vi "GEM_BANK_ARRAY_Flatten.vi"(8 "error in (no error)":errorcluster, 11 "LVBANKARRAY in":refnum<class "GEM_BANK_ARRAY.lvclass">) -> (0 "error out":errorcluster, 2 "Array":u8[](array[numeric]), 3 "LVBANKARRAY out":refnum<class "GEM_BANK_ARRAY.lvclass">)   [LabVIEW 2018, in "feGEM DataPacker.lvlib" / "GEM_BANK_ARRAY.lvclass"]
uses:
  GEM_BANK_ARRAY.lvclass
  GEM_BANK_ARRAY.lvclass/GEM_BANK_ARRAY.ctl
  GEM_BANK.lvclass
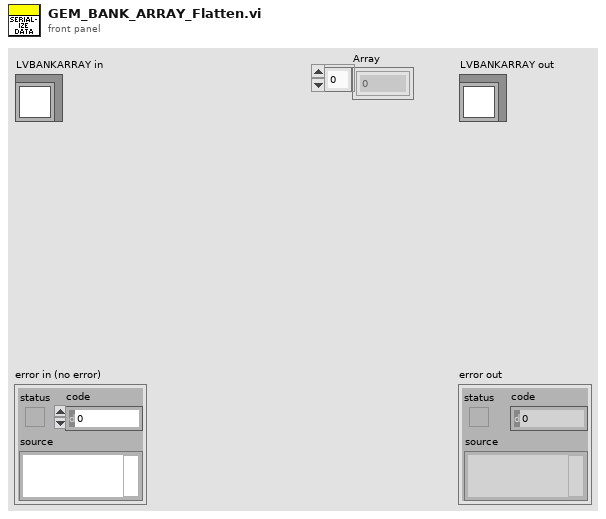
[diagram p1: front panel]
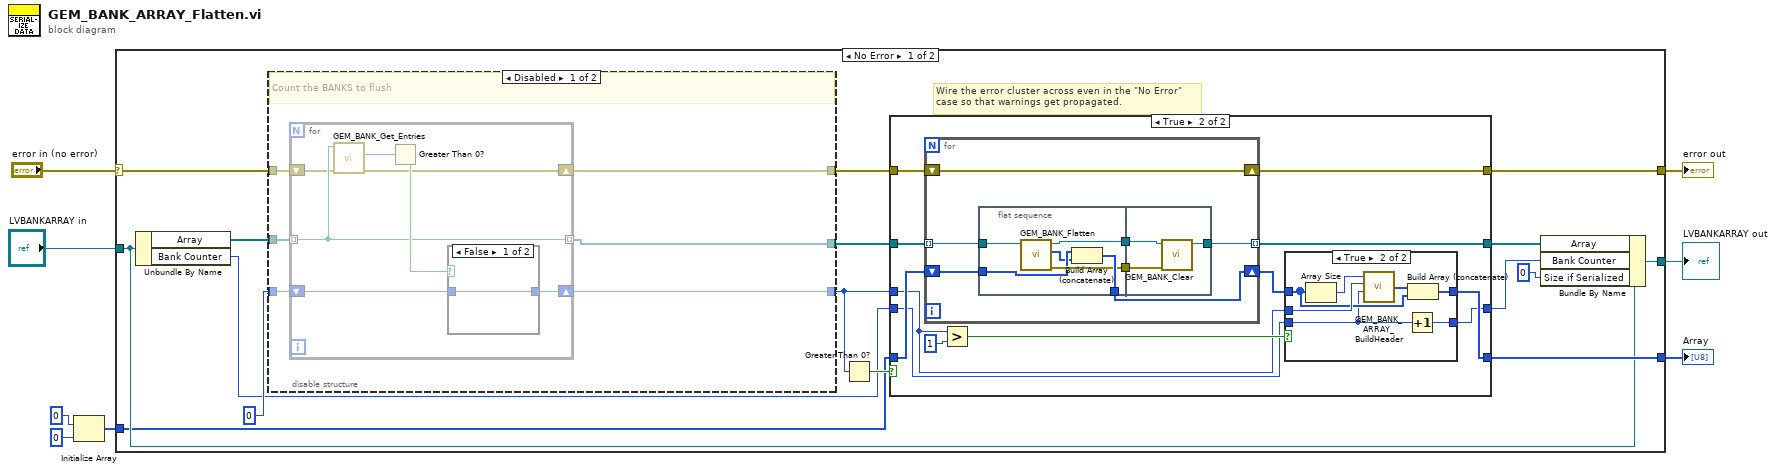
[diagram p0: block diagram]
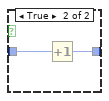
[diagram p2: hidden frame]
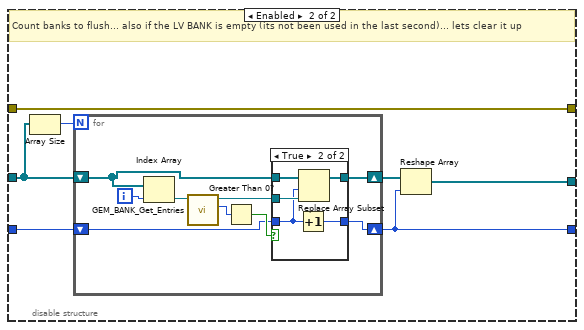
[diagram p3: hidden frame]
diagram:
  n1 = Initialize Array(u8 0 ("element"), 0 ("dimension size")) -> (w4:u8[])
  n2 = case shown="No Error" "error in (no error)" {
    selector: "error in (no error)" -> [w15 w107]
    tunnel: [w13 w107] -> w7
    tunnel: [w18 w106] -> w5
    tunnel: "LVBANKARRAY in" -> [w17 w106]
    tunnel: [w19 w105] -> w1
    tunnel: w4 -> [w16 w105]
    frame No Error {
      # "Wire the error cluster across even in the \"No Error\"\ncase so that warnings get propagated."
      n3 = Unbundle By Name(w17) -> ("Array"=w24:refnum<class "GEM_BANK.lvclass">[], "Bank Counter"=w12:u32)
      n4 = disable-structure shown="Disabled" {
        disable-tunnel: w24 -> [w30 w46]
        disable-tunnel: 0 -> [w29 w42]
        disable-tunnel: [w28 w41] -> w21
        disable-tunnel: [w27 w44] -> w9
        disable-tunnel: w15 -> [w26 w43]
        disable-tunnel: [w25 w43] -> w14
        frame Disabled {
          # "Count the BANKS to flush"
          n5 = for {
            tunnel: w30 -> [w33] mode=indexing
            shift-right: [w34] -> w28
            shift-left: w29 -> [w35]
            tunnel: [w33] -> w27 mode=indexing
            shift-right: [w31] -> w25
            shift-left: w26 -> [w32]
            n6 = call "GEM_BANK_Get_Entries.vi"("error in (no error)"=w32, "LVBANK in"=w33) -> ("error out"=w31:errorcluster, "Count of LVDATA"=w37:i32)  [unwired: 7 in, 1 out]
            n7 = Greater Than 0?(x=w37) -> (x > 0?=w36:bool)
            n8 = case shown="False" w36 {
              tunnel: w35 -> [w38 w40]
              tunnel: [w38 w39] -> w34
              frame False {
              }
              frame True {
                n9 = Increment(x=w40) -> (x+1=w39:i32)
              }
            }
          }
        }
        frame Enabled {
          # "Count banks to flush... also if the LV BANK is empty (its not been used in the last second)... lets clear it up"
          n10 = Array Size(array=w46) -> (size(s)=w47:i32)
          n11 = for {
            N: w47 -> [_]
            shift-right: [w49] -> w41
            shift-left: w42 -> [w50]
            shift-right: [w48] -> w45
            shift-left: w46 -> [w54]
            i -> [w56]
            n12 = Index Array(array=w54, index=w56) -> (element=w55:refnum<class "GEM_BANK.lvclass">)
            n13 = call "GEM_BANK_Get_Entries.vi"("LVBANK in"=w55) -> ("Count of LVDATA"=w53:i32, "LVBANK out"=w51:refnum<class "GEM_BANK.lvclass">)  [unwired: 8 in, 1 out]
            n14 = Greater Than 0?(x=w53) -> (x > 0?=w52:bool)
            n15 = case shown="True" w52 {
              tunnel: w54 -> [w57 w63]
              tunnel: w51 -> [_ w62]
              tunnel: w50 -> [w58 w61]
              tunnel: [w58 w60] -> w49
              tunnel: [w57 w59] -> w48
              frame False {
              }
              frame True {
                n16 = Increment(x=w61) -> (x+1=w60:i32)
                n17 = Replace Array Subset(array=w63, new element=w62, index=w61) -> (w59:refnum<class "GEM_BANK.lvclass">[])
              }
            }
          }
          n18 = Reshape Array(w45, w41) -> (w44:refnum<class "GEM_BANK.lvclass">[])
        }
      }
      n19 = Greater Than 0?(x=w21) -> (x > 0?=w22:bool)
      n20 = case shown="True" w22 {
        tunnel: w21 -> [_ w68]
        tunnel: w9 -> [w67 w77]
        tunnel: [w67 w76] -> w20
        tunnel: w16 -> [w66 w75]
        tunnel: [w66 w74] -> w19
        tunnel: w14 -> [w65 w72]
        tunnel: [w65 w71] -> w13
        tunnel: w12 -> [w64 w70]
        tunnel: [w64 w69] -> w11
        frame False {
        }
        frame True {
          n21 = for {
            tunnel: w77 -> [w86] mode=indexing
            tunnel: [w84] -> w76 mode=indexing
            shift-right: [w82] -> w73
            shift-left: w75 -> [w83]
            shift-right: [w80] -> w71
            shift-left: w72 -> [w80]
            n22 = flat-sequence {
              tunnel: w86 -> [w92]
              tunnel: [w91] -> w85
              tunnel: w83 -> [w88]
              tunnel: [w90] -> w82
              tunnel: [w89] -> w81
              tunnel: w85 -> [w95]
              tunnel: [w94] -> w84
              tunnel: w81 -> [w93]
              frame #0 {
                n23 = call "GEM_BANK_Flatten.vi"("LVBANK in"=w92) -> ("error out"=w89:errorcluster, "output array"=w87:u8[], "LVBANK out"=w91:refnum<class "GEM_BANK.lvclass">)  [unwired: 8 in]
                n24 = Build Array (concatenate)(w88, w87) -> (w90:u8[])
              }
              frame #1 {
                n25 = call "GEM_BANK_Clear.vi"("error in (no error)"=w93, "LVBANK in"=w95) -> ("LVBANK out"=w94:refnum<class "GEM_BANK.lvclass">)  [unwired: 8 in, 1 out]
              }
            }
          }
          n26 = Greater?(x=w68, y=1) -> (0:w78:bool)
          n27 = case shown="True" w78 {
            tunnel: w68 -> [_ w104]
            tunnel: w73 -> [w97 w101]
            tunnel: [w97 w102] -> w74
            tunnel: w70 -> [w96 w99]
            tunnel: [w96 w98] -> w69
            frame False {
            }
            frame True {
              n28 = Array Size(array=w101) -> (size(s)=w100:i32)
              n29 = call "GEM_BANK_ARRAY_BuildHeader.vi"("BANK NUMBER"=w99, "Number of LVBANK entries"=w104, "Size of data bundle"=w100) -> ("output"=w103:u8[])  [unwired: 1 in]
              n30 = Increment(x=w99) -> (x+1=w98:u32)
              n31 = Build Array (concatenate)(w103, w101) -> (w102:u8[])
            }
          }
        }
      }
      n32 = Bundle By Name(cluster=w17, "Array"=w20, "Bank Counter"=w11, "Size if Serialized"=u32 0) -> (w18:refnum<class "GEM_BANK_ARRAY.lvclass">)
    }
    frame Error {
    }
  }
  "error out" <- w7
  "LVBANKARRAY out" <- w5
  "Array" <- w1
